vi "WS1050_FPGA_Init.vi"(8 "error in":errorcluster) -> (0 "error out":errorcluster)   [LabVIEW 2012]
panel:
  # "Initialize AD7747 for Capacitance Measurement Mode"
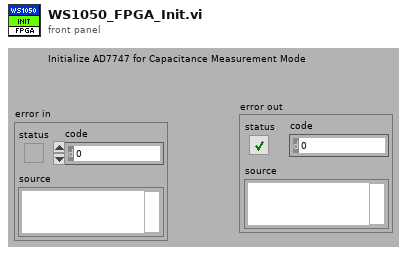
[diagram p1: front panel]
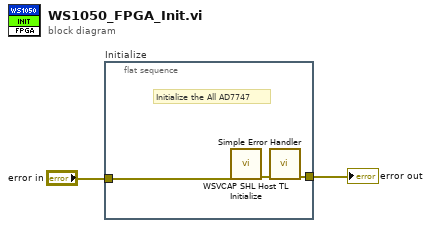
[diagram p0: block diagram]
diagram:
  n1 = flat-sequence "Initialize" {
    tunnel: "error in" -> [w3]
    tunnel: [w4] -> w1
    frame #0 {
      # "Initialize the All AD7747"
      n2 = call "WSVCAP SHL Host TL Initialize.vi"("error in"=w3) -> ("error out"=w5:errorcluster)  [unwired: 14 in]
      n3 = call <vilib>:"Simple Error Handler.vi"("error in (no error)"=w5) -> ("error out"=w4:errorcluster)  [unwired: 4 in, 4 out]
    }
  }
  "error out" <- w1
